vi "Open.vi"(8 "error in (no error)":errorcluster, 10 "Serial Info":T2, 11 "Controller Queue in":T1) -> (0 "error out":errorcluster, 3 "Controller Queue out":T1)   [LabVIEW 2019, in "Controller.lvlib"]
uses:
  Controller.lvlib
  Controller Message Queue.ctl
  Controller Message.ctl
  MDS Command.ctl
  Serial Info.ctl
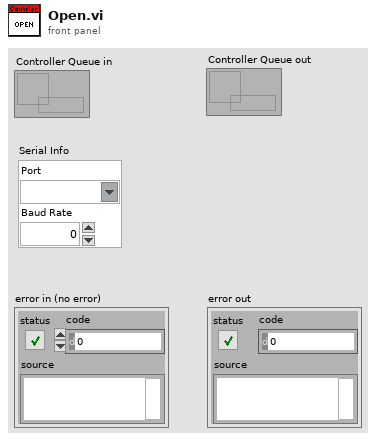
[diagram p1: front panel]
types:
  T1 = typedef "Controller.lvlib/Controller Message Queue.ctl" = refnum<queue>
  T2 = typedef "Controller.lvlib/Serial Info.ctl" = cluster{"Port":refnum<visa-resource-name>, "Baud Rate":u32}
  T3 = typedef "Controller.lvlib/Controller Message.ctl" = cluster{"MDS Command":T4, "Channel":u8, "Value":variant}
  T4 = typedef "Controller.lvlib/MDS Command.ctl" = enum16{"Idle", "Open", "Set VMode", "Set IMode", "Get Frequency", "Set Frequency", "Get Power", "Set Power (dBm)", "Set Power (%)", "Get Switch", "Switch Channel", "Store", "Wait for Prompt", "Wait for State", "Reset", "Error", "Close", "Stop"}
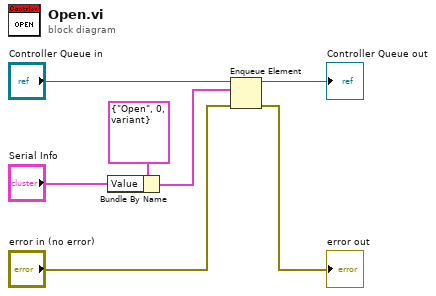
[diagram p0: block diagram]
diagram:
  n1 = Bundle By Name(cluster=T3 {"MDS Command"=enum."Open", "Channel"=0, "Value"=variant} ("Controller Message"), "Value"="Serial Info") -> (w4:T3)
  n2 = Enqueue Element(queue="Controller Queue in", element=w4, error in (no error)="error in (no error)") -> (queue out=→"Controller Queue out":T1, error out=→"error out":errorcluster)  [unwired: 1 in, 1 out]
